vi "Demo.vi"() -> ()   [LabVIEW 2017]
uses:
  ctl/LVDataSetting.ctl
  LVData.lvclass
panel:
  in  "?":enum32{"CONFIG", "MEASUREMENT"}(tab)
  in  "File Path Control":path
  in  "Setting1":T1
  in  "milliseconds to wait":u32
  in  "Activate":bool
  out "error out":errorcluster
  in  "stop":bool
  out "Graph 1":T2(graph) caption="XY Graph"
  out "Last Data acquired":dbl[](array[numeric])
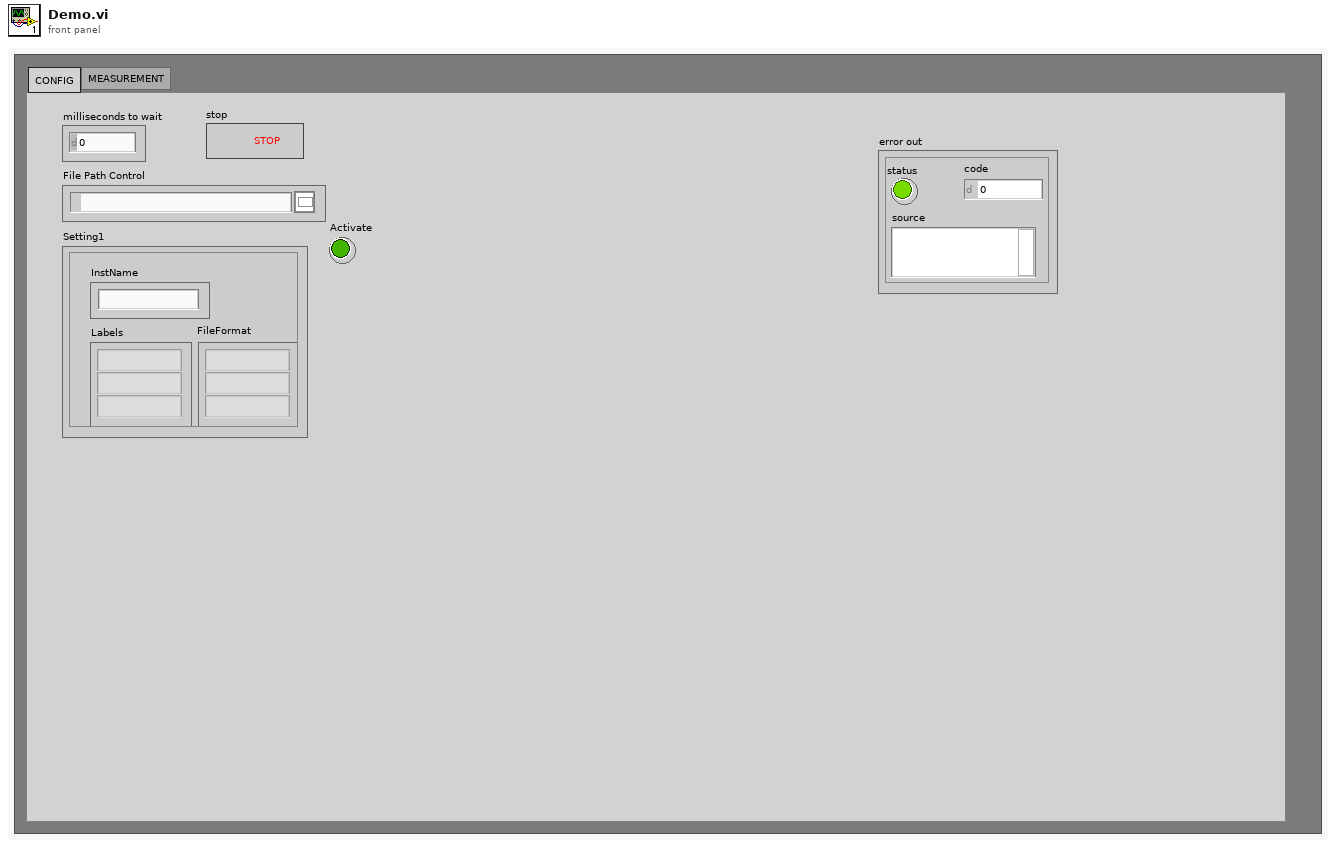
[diagram p1: front panel]
types:
  T1 = typedef "LVDataSetting.ctl" = cluster{"Labels":string[], "InstName":string, "FileFormat":string[]}
  T2 = cluster{"TimeArray":timestamp[], "DataArray":dbl[]}[]
  T3 = cluster{"TimeArray":timestamp[], "DataArray":dbl[]}
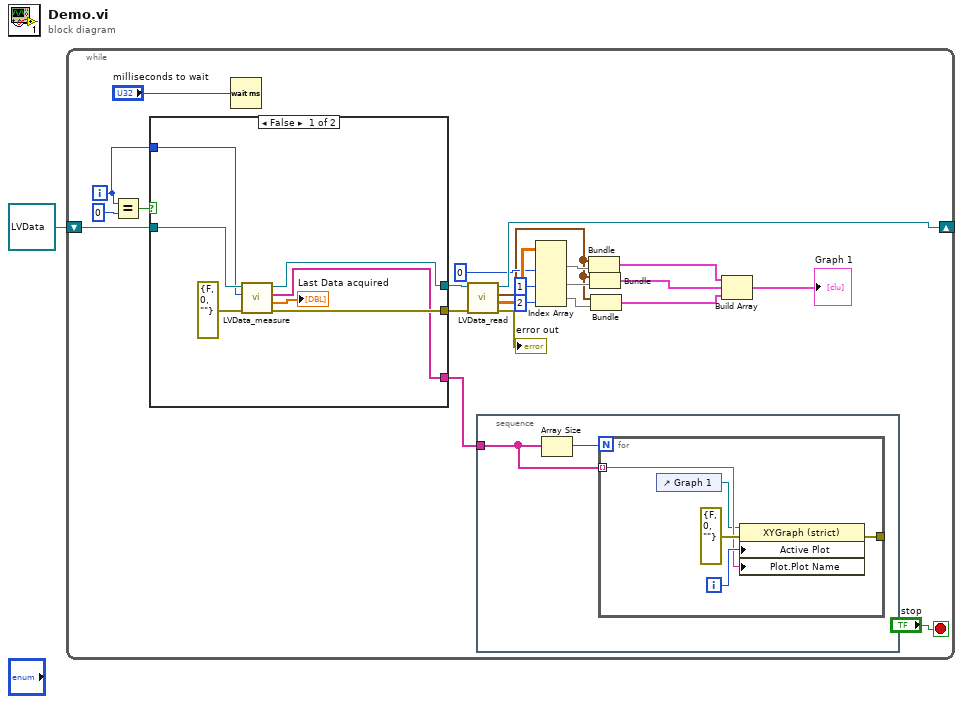
[diagram p0: block diagram]
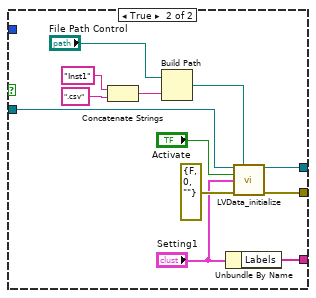
[diagram p2: hidden frame]
diagram:
  n1 = while {
    shift-right: [w18] -> _
    shift-left: refnum<class "LVData.lvclass"> refnum ("LVData.lvclass") -> [w24]
    i -> [w2]
    stop <- "stop" stop-if-true
    n2 = Equal?(x=w2, y=0) -> (x = y?=w21:bool)
    n3 = case shown="False" w21 {
      tunnel: w24 -> [w38 w50]
      tunnel: [w37 w47] -> w17
      tunnel: [w35 w41] -> w19
      tunnel: [w33 w39] -> w12
      tunnel: w2 -> [w32 _]
      frame False {
        n4 = call-dynamic "LVData_measure.vi"("error in (no error)"=errorcluster {"status"=FALSE, "code"=0, "source"=""}, "index"=w32, "LVData in"=w38) -> ("error out"=w37:errorcluster, "Data acquired"=→"Last Data acquired":dbl[], "Labels"=w33:string[], "LVData out"=w35:refnum<class "LVData.lvclass">)  [unwired: 5 in]
      }
      frame True {
        n5 = Concatenate Strings("Inst1" ("name or relative path"), ".csv" ("string")) -> (w43:string)
        n6 = Build Path(base path="File Path Control", name or relative path=w43) -> (appended path=w42:path)
        n7 = Unbundle By Name("Setting1") -> ("Labels"=w39:string[])
        n8 = call-dynamic "LVData_initialize.vi"("LVData in"=w50, "FilePath"=w42, "Activate"="Activate", "Setting"="Setting1", "error in (no error)"=errorcluster {"status"=FALSE, "code"=0, "source"=""}) -> ("LVData out"=w41:refnum<class "LVData.lvclass">, "error out"=w47:errorcluster)  [unwired: 9 in]
      }
    }
    n9 = Wait (ms)(milliseconds to wait="milliseconds to wait") -> ()  [unwired: 1 out]
    n10 = call "LVData_read.vi"("error in (no error)"=w17, "LVData in"=w19) -> ("error out"=→"error out":errorcluster, "DataArray"=w15:dbl[][], "TimeArray"=w8:timestamp[], "LVData out"=w18:refnum<class "LVData.lvclass">)  [unwired: 5 in, 1 out]
    n11 = stacked-sequence {
      tunnel: w12 -> [w25]
      frame #0 {
        n12 = Array Size(array=w25) -> (size(s)=w26:i32)
        n13 = for {
          N: w26 -> [_]
          tunnel: [w29] -> _
          tunnel: w25 -> [w28] mode=indexing
          i -> [w31]
          n14 = control-ref of="Graph 1"() -> (w27:refnum<vi>)
          n15 = property class="XYGraph (strict)"(reference=w27, error in=errorcluster {"status"=FALSE, "code"=0, "source"=""} ("error in (no error)"), "Active Plot"=w31, "Plot.Plot Name"=w28) -> (error out=w29:errorcluster)  [unwired: 1 out]
        }
      }
    }
    n16 = Index Array(array=w15, index (col) #1=0 ("index"), index (col) #2=1 ("index (col)"), index (col) #3=2 ("index (col)")) -> (element #1=w13:dbl[], element #2=w9:dbl[], element #3=w7:dbl[])  [unwired: 3 in]
    n17 = Bundle("TimeArray"=w8, "DataArray"=w13) -> (w6:T3)  [unwired: 1 in]
    n18 = Bundle("TimeArray"=w8, "DataArray"=w9) -> (w5:T3)  [unwired: 1 in]
    n19 = Bundle("TimeArray"=w8, "DataArray"=w7) -> (w4:T3)  [unwired: 1 in]
    n20 = Build Array(w6, w5, w4) -> (→"Graph 1":T2)
  }
